vi "Settings_Config.vi"(11 "DataCluster in":T1={"Core"={"Current VI Reference"=refnum, "Close Panel on Exit?"=FALSE, "Exit"=FALSE}, "Connections"={"Arduino"={"VISA"="", "Data Feed"="", "Connected"=FALSE}, "Ready"=FALSE}, "Files"={"Path"=path "", "Filename"="", "File List"=1, "Buffer"={"Buffer"=refnum, "Size"=1}, "Downloading"=FALSE}}) -> (3 "DataCluster out":T1={"Core"={"Current VI Reference"=refnum, "Close Panel on Exit?"=FALSE, "Exit"=FALSE}, "Connections"={"Arduino"={"VISA"="", "Data Feed"="", "Connected"=FALSE}, "Ready"=FALSE}, "Files"={"Path"=path "", "Filename"="", "File List"=1, "Buffer"={"Buffer"=refnum, "Size"=1}, "Downloading"=FALSE}})   [LabVIEW 2022 SP3]
uses:
  DataCluster.ctl
panel:
  in  "Sample Volume":dbl=1.0 min=0.0 max=500.0 format="%#_g µL"
  in  "Sample Rate":i32=20 min=20 max=240 step=1 format="%.0f Samples/min"
  in  "Target Temperature":dbl=1.0 min=-30.0 max=30.0 step=0.5 format="%#_g °C"
  in  "OK":bool
  in  "Cancel":bool
  in  "Temperature Gradient":dbl=1.0 min=-100.0 max=100.0 step=0.1 format="%#_g °C/min"
  in  "Notes":string
  in  "Operator":string
  in  "Label":string
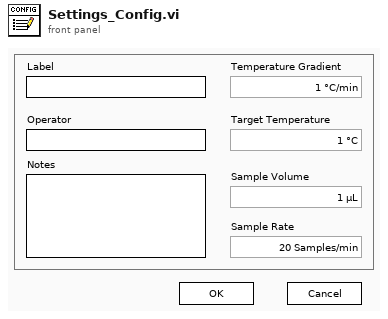
[diagram p1: front panel]
types:
  T1 = typedef "DataCluster.ctl" = cluster{"Core":cluster{"Current VI Reference":refnum<vi>, "Close Panel on Exit?":bool, "Exit":bool}, "Connections":cluster{"Arduino":cluster{"VISA":refnum<visa-resource-name>, "Data Feed":string, "Connected":bool}, "Ready":bool}, "Files":cluster{"Path":path, "Filename":string, "File List":i32, "Buffer":cluster{"Buffer":refnum<queue>, "Size":i32}, "Downloading":bool}}
  T2 = enum8{"Enabled", "Disabled", "Disabled and Grayed Out"}
  T3 = cluster{"Label":string, "Operator":string, "Notes":string, "TempGrad":dbl, "TargetTemp":dbl, "Sample Volume":dbl}
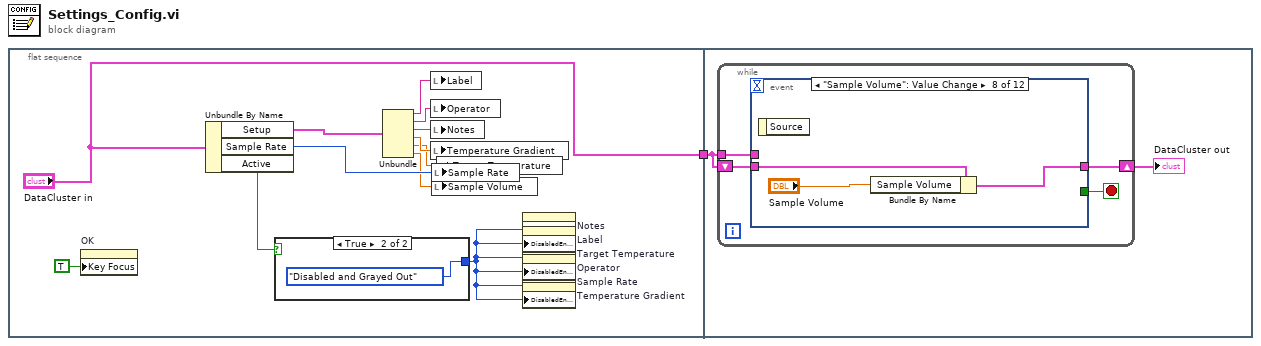
[diagram p0: block diagram]
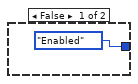
[diagram p2: hidden frame]
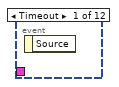
[diagram p3: hidden frame]
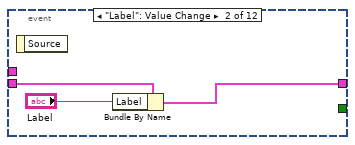
[diagram p4: hidden frame]
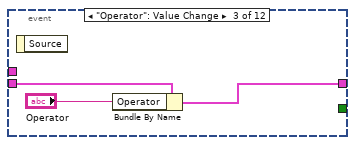
[diagram p5: hidden frame]
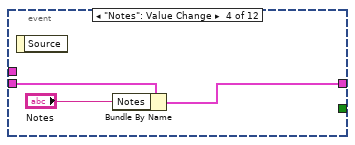
[diagram p6: hidden frame]
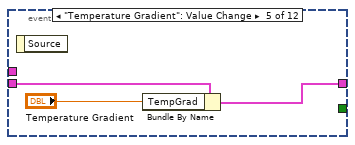
[diagram p7: hidden frame]
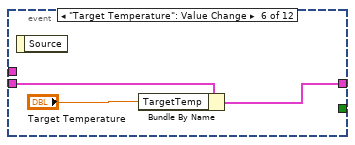
[diagram p8: hidden frame]
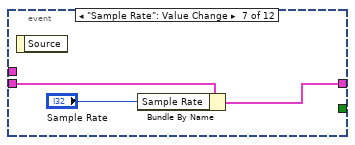
[diagram p9: hidden frame]
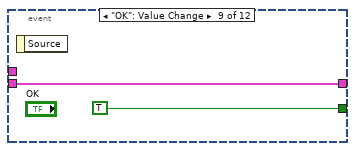
[diagram p10: hidden frame]
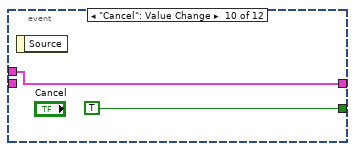
[diagram p11: hidden frame]
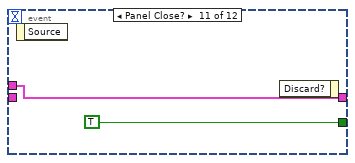
[diagram p12: hidden frame]
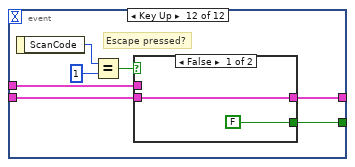
[diagram p13: hidden frame]
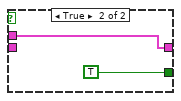
[diagram p14: hidden frame]
diagram:
  n1 = flat-sequence {
    tunnel: ["DataCluster in"] -> w1
    tunnel: w1 -> [w17]
    frame #0 {
      n2 = property on="OK" class="Bool"("Key Focus"=TRUE) -> ()  [unwired: 2 in, 2 out]
      n3 = Unbundle By Name("DataCluster in") -> ("Setup"=w13:T3, "Sample Rate"=w5:i32, "Active"=w6:bool)
      n4 = case shown="True" w6 {
        tunnel: [T2."Enabled" ("Disabled") T2."Disabled and Grayed Out" ("Disabled")] -> w2
        frame False {
        }
        frame True {
        }
      }
      n5 = Unbundle(w13) -> ("Label"=w12:string, "Operator"=w8:string, "Notes"=w7:string, "TempGrad"=w11:dbl, "TargetTemp"=w3:dbl, "Sample Volume"=w4:dbl)
      n6 = local write "Label"(w12) -> ()
      n7 = local write "Operator"(w8) -> ()
      n8 = local write "Notes"(w7) -> ()
      n9 = local write "Temperature Gradient"(w11) -> ()
      n10 = local write "Sample Rate"(w5) -> ()
      n11 = local write "Sample Volume"(w4) -> ()
      n12 = local write "Target Temperature"(w3) -> ()
      n13 = property on="Notes" class="Str"("DisabledEnum"=w2) -> ()  [unwired: 2 in, 2 out]
      n14 = property on="Label" class="Str"("DisabledEnum"=w2) -> ()  [unwired: 2 in, 2 out]
      n15 = property on="Target Temperature" class="DigNum (strict)"("DisabledEnum"=w2) -> ()  [unwired: 2 in, 2 out]
      n16 = property on="Operator" class="Str"("DisabledEnum"=w2) -> ()  [unwired: 2 in, 2 out]
      n17 = property on="Sample Rate" class="DigNum (strict)"("DisabledEnum"=w2) -> ()  [unwired: 2 in, 2 out]
      n18 = property on="Temperature Gradient" class="DigNum (strict)"("DisabledEnum"=w2) -> ()  [unwired: 2 in, 2 out]
    }
    frame #1 {
      n19 = while {
        shift-right: [w21] -> w16
        shift-left: w17 -> [w20]
        tunnel: w17 -> [w19]
        stop <- w18 stop-if-true
        n20 = event shown="[7] \"Sample Volume\": Value Change" {
          selector: _ -> [_ _ _ _ _ _ _ _ _ _ _ _]
          dyn-events: _ -> [_ _ _ _ _ _ _ _ _ _ _ _]
          timeout: _ -> [_ _ _ _ _ _ _ _ _ _ _ _]
          tunnel: w20 -> [_ w24 w27 w30 w33 w36 w39 w42 w44 _ _ w49]
          tunnel: [_ w23 w26 w29 w32 w35 w38 w41 w44 w46 w48 w51] -> w21
          tunnel: w19 -> [_ _ _ _ _ _ _ _ _ w46 w48 w50]
          tunnel: [_ _ _ _ _ _ _ _ TRUE TRUE TRUE w55] -> w18
          event Timeout {
            n21 = event-data() -> ()  [unwired: 1 in, 1 out]
          }
          event "Label": Value Change {
            n22 = event-data() -> ()  [unwired: 1 in, 1 out]
            n23 = Bundle By Name(cluster=w24, "Label"="Label") -> (w23:T1)
          }
          event "Operator": Value Change {
            n24 = event-data() -> ()  [unwired: 1 in, 1 out]
            n25 = Bundle By Name(cluster=w27, "Operator"="Operator") -> (w26:T1)
          }
          event "Notes": Value Change {
            n26 = event-data() -> ()  [unwired: 1 in, 1 out]
            n27 = Bundle By Name(cluster=w30, "Notes"="Notes") -> (w29:T1)
          }
          event "Temperature Gradient": Value Change {
            n28 = event-data() -> ()  [unwired: 1 in, 1 out]
            n29 = Bundle By Name(cluster=w33, "TempGrad"="Temperature Gradient") -> (w32:T1)
          }
          event "Target Temperature": Value Change {
            n30 = event-data() -> ()  [unwired: 1 in, 1 out]
            n31 = Bundle By Name(cluster=w36, "TargetTemp"="Target Temperature") -> (w35:T1)
          }
          event "Sample Rate": Value Change {
            n32 = event-data() -> ()  [unwired: 1 in, 1 out]
            n33 = Bundle By Name(cluster=w39, "Sample Rate"="Sample Rate") -> (w38:T1)
          }
          event "Sample Volume": Value Change {
            n34 = event-data() -> ()  [unwired: 1 in, 1 out]
            n35 = Bundle By Name(cluster=w42, "Sample Volume"="Sample Volume") -> (w41:T1)
          }
          event "OK": Value Change {
            n36 = event-data() -> ()  [unwired: 1 in, 1 out]
          }
          event "Cancel": Value Change {
            n37 = event-data() -> ()  [unwired: 1 in, 1 out]
          }
          event Panel Close? {
            n38 = event-data() -> ()  [unwired: 1 in, 1 out]
            n39 = event-data() -> ()  [unwired: 2 in, 1 out]
          }
          event Key Up {
            # "Escape pressed?"
            n40 = event-data() -> ("ScanCode"=w54:i16)  [unwired: 1 in]
            n41 = Equal?(x=w54, y=i16 1) -> (x = y?=w52:bool)
            n42 = case shown="False" w52 {
              tunnel: [FALSE TRUE] -> w55
              tunnel: [w57 w58] -> w51
              tunnel: w50 -> [_ w58]
              tunnel: w49 -> [w57 _]
              frame False {
              }
              frame True {
              }
            }
          }
        }
      }
      "DataCluster out" <- w16
    }
  }
